vi "Read UE_From1PLOT.vi"(8 "error in (no error)":errorcluster, 11 "StokePlotHandle in":refnum<class "BjusticePlotHandle.lvclass">) -> (0 "error out":errorcluster, 2 "UE:From1PLOT":refnum<user-event>, 3 "StokePlotHandle out":refnum<class "BjusticePlotHandle.lvclass">)   [LabVIEW 2021, in "BjusticePlotHandle.lvclass"]
uses:
  BjusticePlotHandle.lvclass
  1PLOT to MPLOT UE.ctl
  1PLOT to MPLOT type.ctl
  BjusticePlotHandle.lvclass/BjusticePlotHandle.ctl
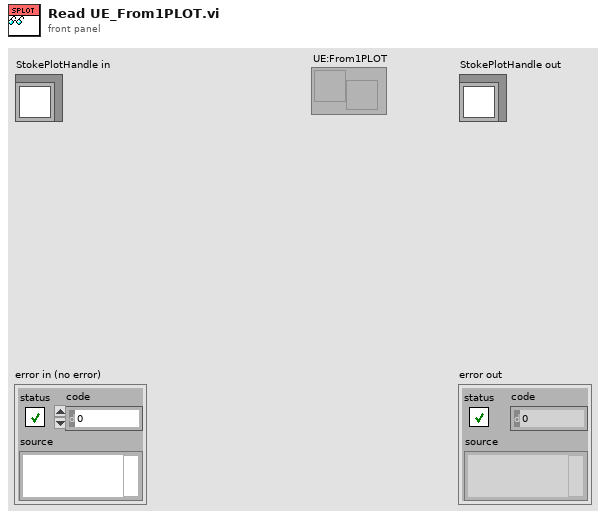
[diagram p1: front panel]
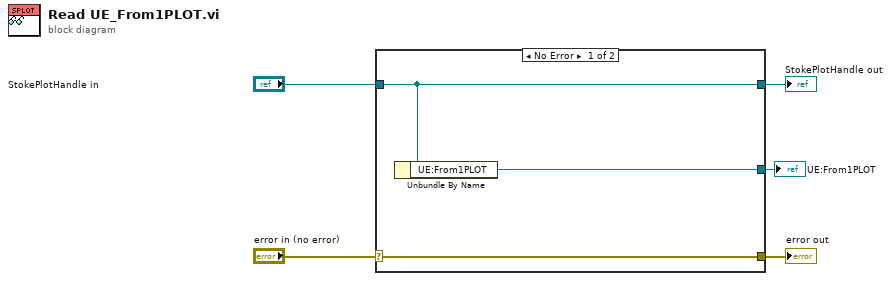
[diagram p0: block diagram]
diagram:
  n1 = case shown="No Error" "error in (no error)" {
    selector: "error in (no error)" -> [w8 w9]
    tunnel: [w8 w9] -> w4
    tunnel: [w7 w10] -> w2
    tunnel: "StokePlotHandle in" -> [w7 w10]
    tunnel: [w6 _] -> w1
    frame No Error {
      n2 = Unbundle By Name(w7) -> ("UE:From1PLOT"=w6:refnum<user-event>)
    }
    frame Error {
    }
  }
  "error out" <- w4
  "StokePlotHandle out" <- w2
  "UE:From1PLOT" <- w1
